vi "CSM - Mark As Chain Module.vi"(6 "Order":i32, 9 "CSM Name":string="Chain") -> (2 "CSM Name (Marked As Chain)":string)   [LabVIEW 2017, in "Communicable State Machine.lvlib"]
doc: "### CSM - Mark As Chain Module.vi\n\n[!WARNING] This set of functions has not been fully verified, please use with caution.\n\n> Ref: CSM Chain of Responsibility Mode\n> Ref: Name Concatenation API\n\n-- <b>Controls</b> --\n- <b>CSM Name</b>: CSM module name\n- <b>Order</b>: Order in the chain of responsibility mode\n\n-- <b>Indicators</b> --\n- <b>CSM Name (marked as Chain)</b>: CSM module name with \"$\" mark"
uses:
  Communicable State Machine.lvlib
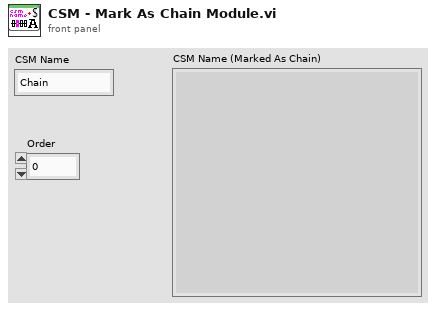
[diagram p1: front panel]
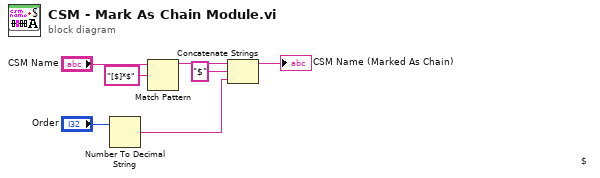
[diagram p0: block diagram]
diagram:
  # "$"
  n1 = Number To Decimal String(number="Order") -> (decimal integer string=w1:string)  [unwired: 1 in]
  n2 = Match Pattern(string="CSM Name", regular expression="[$]*$") -> (before substring=w5:string)  [unwired: 1 in, 3 out]
  n3 = Concatenate Strings(w5, "$" ("string"), w1) -> (→"CSM Name (Marked As Chain)":string)
